vi "Voltage input PID.vi"() -> ()   [LabVIEW 2019]
uses:
  <vilib>/addons/control/pid/autopid.llb/PID Autotuning Design (Auto).vi
  <vilib>/measure/NI_MABase.lvlib
  <vilib>/addons/control/pid/NI_PID_autopid.lvlib
panel:
  out "Process variable and Setpoint":cluster{"initial PV":dbl, "SP:":dbl}(graph)
  in  "reset signal":bool
  in  "offset":dbl=5.0 format="%0.2p"
  in  "sampling info":cluster{"Fs":dbl, "#s":dbl}={"Fs"=1000.0, "#s"=1000.0} {"Fs" format="%.2p"}
  in  "phase":dbl format="%.2p"
  in  "amplitude":dbl=5.0 format="%0.2p"
  in  "frequency":dbl=0.01 format="%#.6g"
  in  "signal type":T1(ring)
  out "Voltage input Error":waveform(dbl)(graph)
  out "Valve input voltage":dbl(graph)
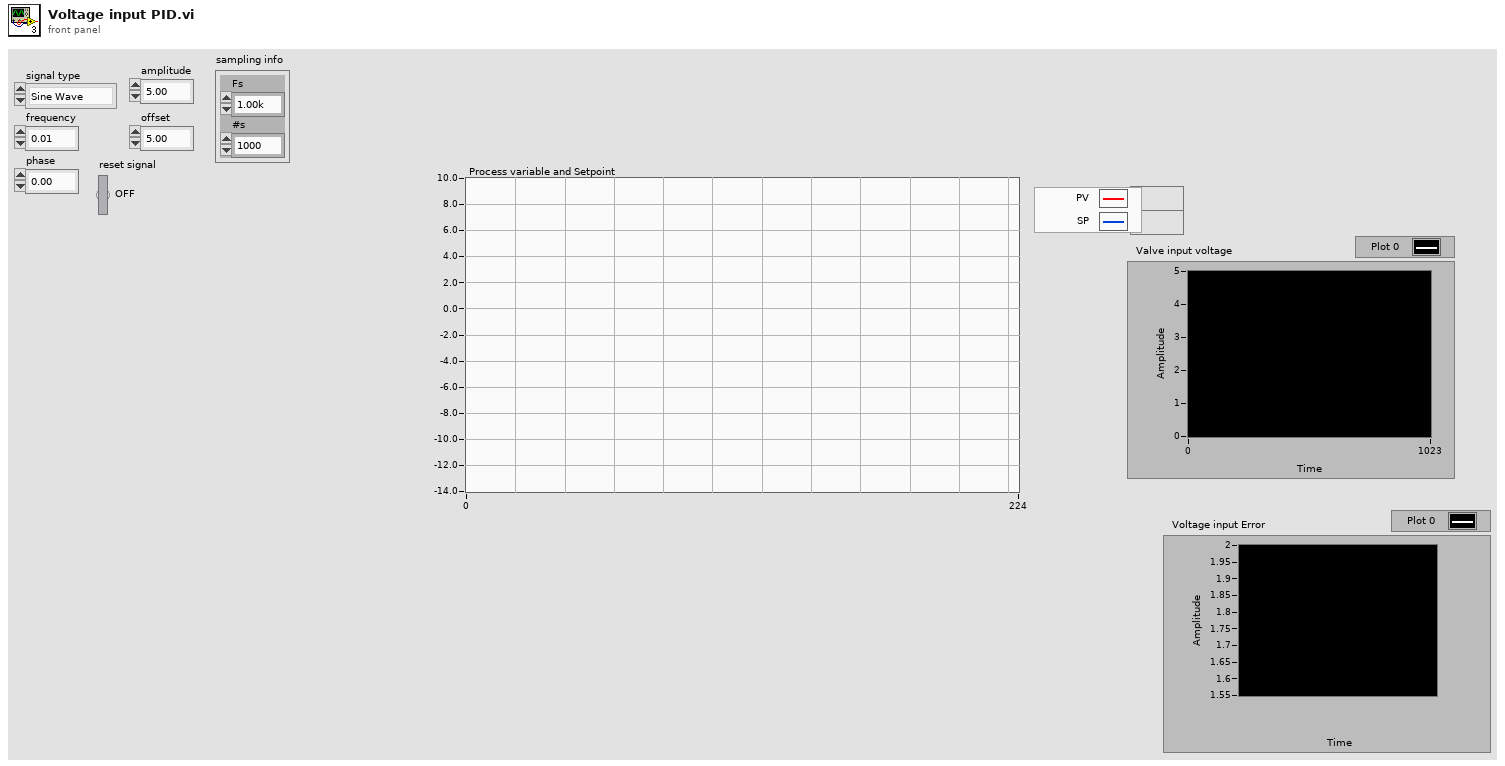
[diagram p1: front panel]
types:
  T1 = enum16{"Sine Wave", "Triangle Wave", "Square Wave", "Sawtooth Wave"}
  T2 = cluster{"Voltage":dbl, "signal out":waveform(dbl)}
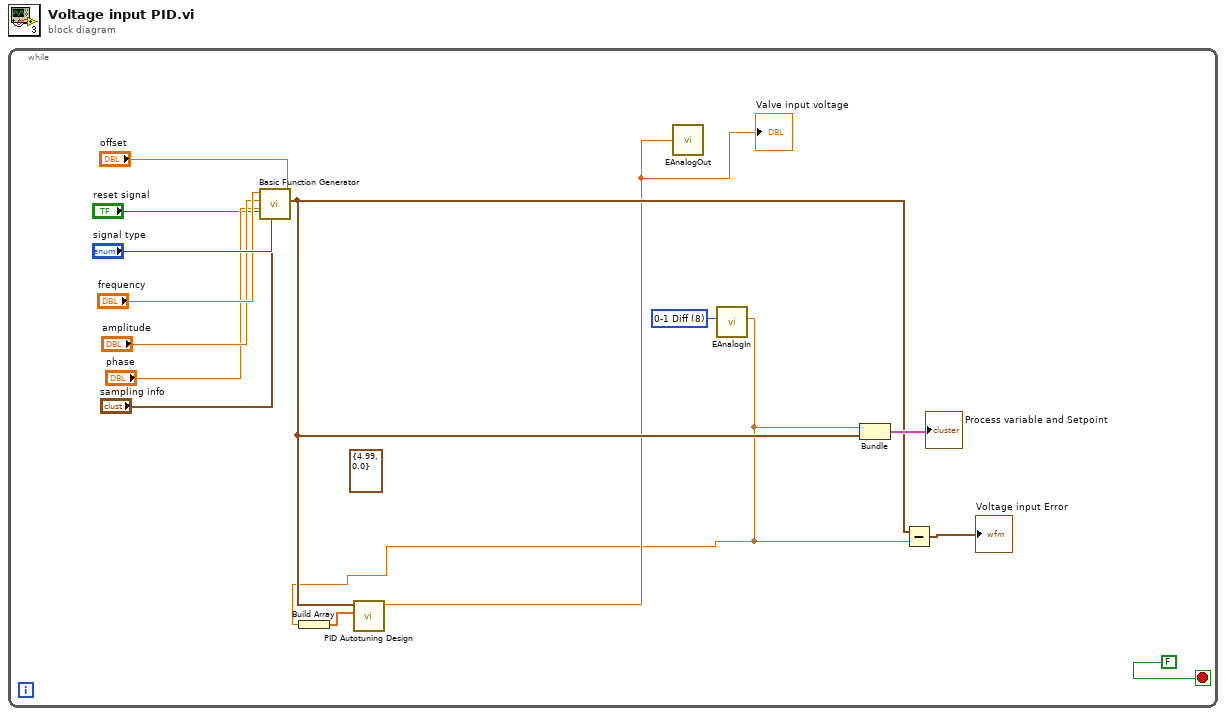
[diagram p0: block diagram]
diagram:
  n1 = while {
    stop <- FALSE stop-if-true
    (unwired) cluster{"output high":dbl, "output low":dbl} {"output high"=4.99, "output low"=0.0} ("output range")
    w15 = u16 8 items=["0 SE (+/-10V)", "1 SE (+/-10V)", "2 SE (+/-10V)", "3 SE (+/-10V)", "4 SE (+/-10V)", "5 SE (+/-10V)", "6 SE (+/-10V)", "7 SE (+/-10V)", "0-1 Diff", "2-3 Diff", "4-5 Diff", "6-7 Diff"] ("Channel")
    n2 = call <vilib>:"Basic Function Generator.vi"("offset"="offset", "reset signal"="reset signal", "sampling info"="sampling info", "signal type"="signal type", "phase"="phase", "amplitude"="amplitude", "frequency"="frequency") -> ("signal out"=w4:waveform(dbl))  [unwired: 2 in, 2 out]
    n3 = call <vilib>:"EAnalogIn.vi"("Channel"=w15) -> ("Voltage"=w1:dbl)  [unwired: 6 in, 4 out]
    n4 = Build Array(w1) -> (w2:dbl[])
    n5 = call-poly <vilib>:"PID Autotuning Design.vi"("Response signal"=w2, "Stimulus signal"=w4) -> ("stimulus operating point"=w3:dbl)  [unwired: 6 in, 3 out]
    "Valve input voltage" <- w3
    n6 = call <vilib>:"EAnalogOut.vi"("Analog Output 0 [volts]"=w3) -> ()  [unwired: 13 in, 2 out]
    n7 = Bundle("Voltage"=w1, "signal out"=w4) -> (→"Process variable and Setpoint":T2)  [unwired: 1 in]
    n8 = Subtract(x=w4, y=w1) -> (x-y=→"Voltage input Error":waveform(dbl))
  }
